vi "findleftmostbitI16x.vi"(1 "x":i16 format="%b") -> (0 "index":i16)   [LabVIEW 2018, in "posit.lvlib"]
uses:
  posit.lvlib
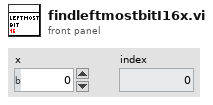
[diagram p1: front panel]
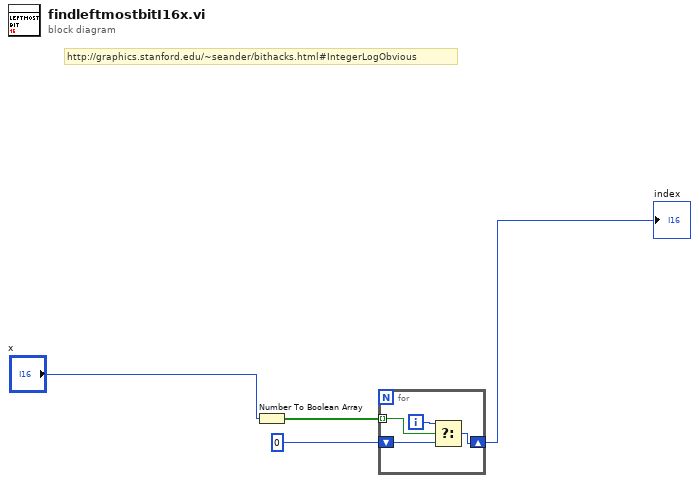
[diagram p0: block diagram]
diagram:
  # "http://graphics.stanford.edu/~seander/bithacks.html#IntegerLogObvious"
  n1 = Number To Boolean Array(number="x") -> (Boolean array=w3:bool[])
  n2 = for {
    tunnel: w3 -> [w8] mode=indexing
    shift-right: [w5] -> w2
    shift-left: 0 -> [w6]
    i -> [w7]
    n3 = Select(t=w7, s=w8, f=w6) -> (s? t:f=w5:i32)
  }
  "index" <- w2
